vi "GetClassImplementationTypeDefNames.vi"(8 "error in (no error)":errorcluster, 11 "ClassReaderNative in":refnum<class "ClassReaderGOOP300.lvclass">) -> (0 "error out":errorcluster, 2 "ImplementationMethodNames":string[](array[string]), 3 "ClassReaderNative out":refnum<class "ClassReaderGOOP300.lvclass">)   [LabVIEW 2020, in "ClassReaderGOOP300.lvclass"]
uses:
  <resource>/Framework/Providers/Open_GDS/ClassProviders/Provider_EndevoGOOP300/ClassReaderGOOP300_class/ClassReaderGOOP300.lvclass
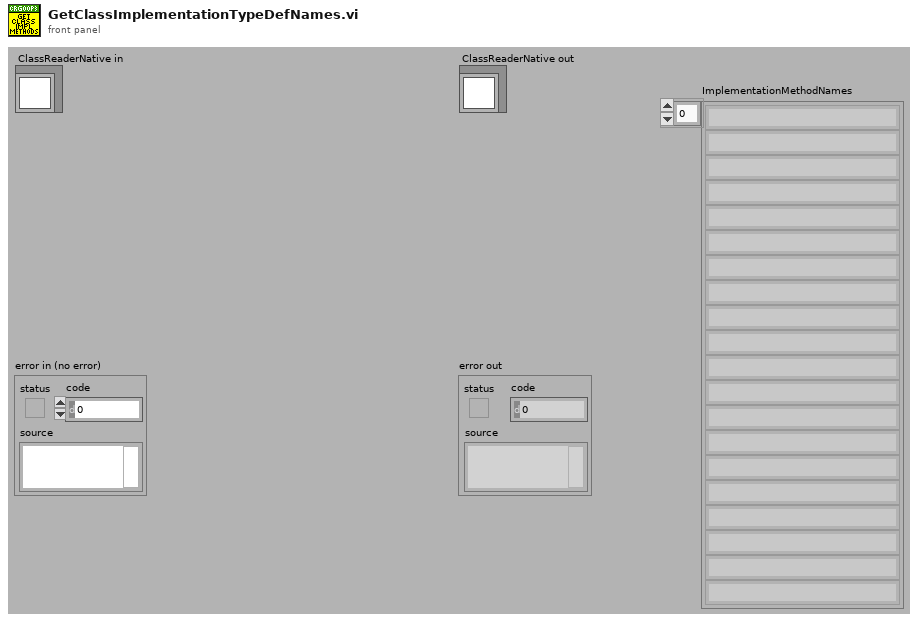
[diagram p1: front panel]
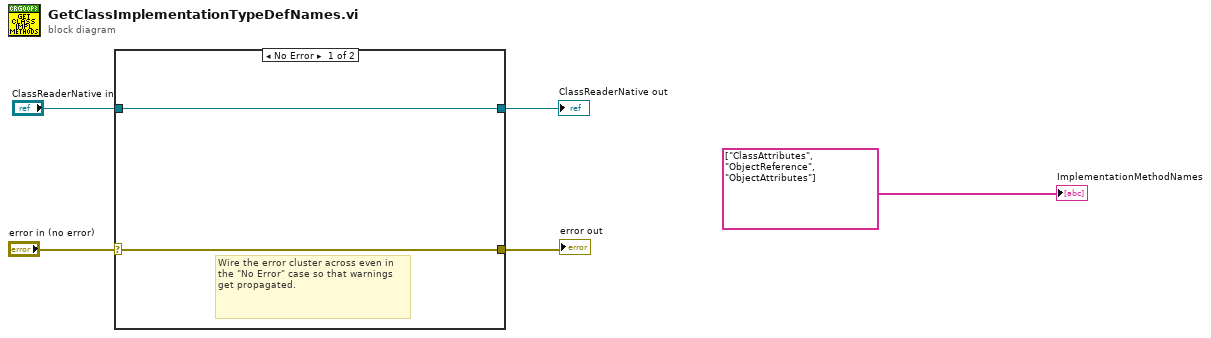
[diagram p0: block diagram]
diagram:
  n1 = case shown="No Error" "error in (no error)" {
    selector: "error in (no error)" -> [w6 w9]
    tunnel: [w6 w9] -> w4
    tunnel: [w7 w8] -> w2
    tunnel: "ClassReaderNative in" -> [w7 w8]
    frame No Error {
      # "Wire the error cluster across even in the \"No Error\" case so that warnings get propagated."
    }
    frame Error {
    }
  }
  "error out" <- w4
  "ClassReaderNative out" <- w2
  "ImplementationMethodNames" <- string[] ["ClassAttributes", "ObjectReference", "ObjectAttributes"] ("ImplementationMethodNames")
